vi "Write Tektronix Configuration.vi"(8 "error in (no error)":errorcluster, 10 "Tektronix Configuration":T1={"Channel"=0, "Number of averages"=4096, "Input impedace"=enum."1 M Ohm", "Vertical coupling"=enum."AC"}, 11 "Tektronix Driver in":refnum<class "Tektronix 7000 Driver.lvclass">) -> (0 "error out":errorcluster, 3 "Tektronix Driver out":refnum<class "Tektronix 7000 Driver.lvclass">)   [LabVIEW 2020, in "Tektronix 7000 Driver.lvclass"]
uses:
  Tektronix 7000 Driver.lvclass
  Tektronix Configuration.ctl
  Tektronix 7000 Driver.lvclass/Tektronix 7000 Driver.ctl
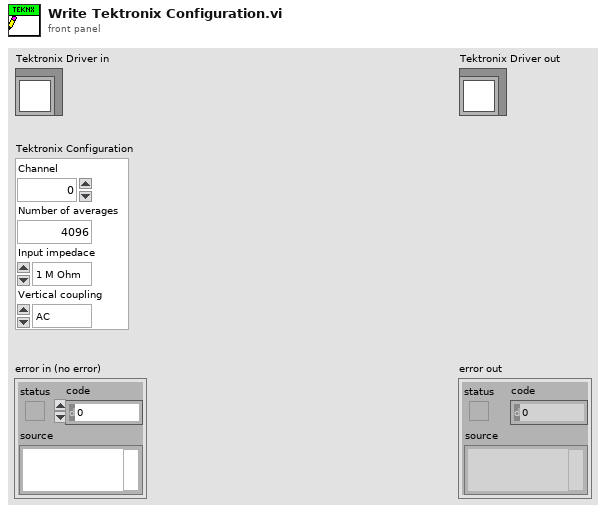
[diagram p1: front panel]
types:
  T1 = typedef "Tektronix Configuration.ctl" = cluster{"Channel":i32, "Number of averages":i32, "Input impedace":enum16{"1 M Ohm", "50 Ohm"}, "Vertical coupling":enum16{"AC", "DC", "Ground"}}
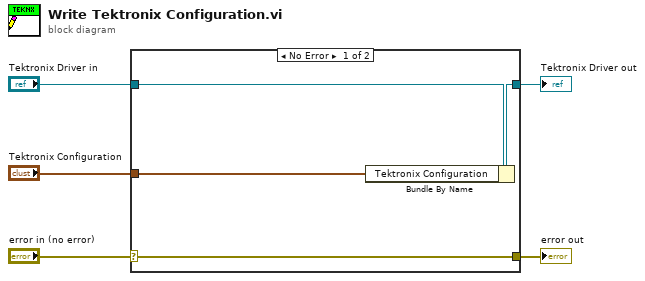
[diagram p0: block diagram]
diagram:
  n1 = case shown="No Error" "error in (no error)" {
    selector: "error in (no error)" -> [w9 w10]
    tunnel: [w9 w10] -> w4
    tunnel: [w7 w11] -> w2
    tunnel: "Tektronix Driver in" -> [w8 w11]
    tunnel: "Tektronix Configuration" -> [w6 _]
    frame No Error {
      n2 = Bundle By Name(cluster=w8, "Tektronix Configuration"=w6) -> (w7:refnum<class "Tektronix 7000 Driver.lvclass">)
    }
    frame Error {
    }
  }
  "error out" <- w4
  "Tektronix Driver out" <- w2
